vi "http get last error.vi"(8 "error in (no error)":errorcluster, 10 "buf_len":i32, 11 "buf_ptr":string) -> (0 "error out":errorcluster, 2 "function return":i32, 3 "buf_ptr out":string)   [LabVIEW 2020, in "reqwest-labview.lvlib"]
doc: "int http_get_last_error(unsigned char *buf_ptr,\n int buf_len);"
uses:
  reqwest-labview.lvlib
  reqwest_labview_64.dll
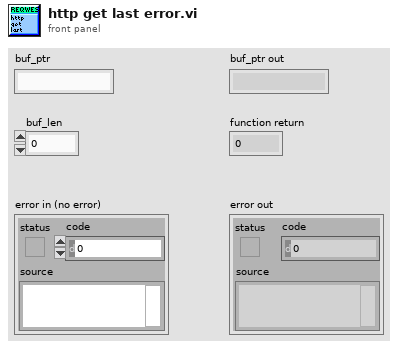
[diagram p1: front panel]
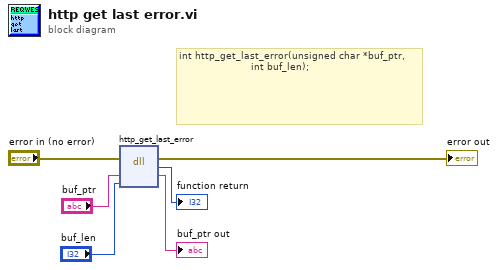
[diagram p0: block diagram]
diagram:
  # "int http_get_last_error(unsigned char *buf_ptr,\n                        int buf_len);"
  n1 = dll-call lib="C:/code/reqwest-labview/lv-src/shared-library/reqwest_labview_*.*" fn="http_get_last_error"(error in="error in (no error)", "buf_ptr"="buf_ptr", "buf_len"="buf_len") -> (error out=→"error out":errorcluster, "return type"=→"function return":i32, "buf_ptr"=→"buf_ptr out":string)  [unwired: 3 in, 1 out]
